vi "Invert if in Avoid Zone.vi"(7 "Avoid Zone (Unit Circle)":T4, 11 "Set Values":T1 {"Angle" scale format="%.3f"; "Velocity" scale=-1.0..1.0 scale format="%.1f"}) -> (2 "In Avoid Zone":bool, 3 "Set Values Out":T1 {"Angle" scale format="%.3f"; "Velocity" scale=-1.0..1.0 scale format="%.1f"})   [LabVIEW 2023, in "TShirtWork-SwerveDrive_ACT_ts.lvlib"]
uses:
  TShirtWork-SwerveDrive_ACT_ts.lvlib
  Shared Code/TypeDefs/Level_Velocity plus-minus 1.ctl
  Shared Code/TypeDefs/Dial_Compase heading unit circle CCW positive.ctl
  Shared Code/TypeDefs/Cluster_Module Velocity-Direction-Rotations.ctl
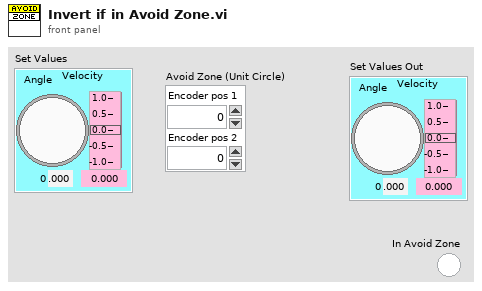
[diagram p1: front panel]
types:
  T1 = typedef "Cluster_Module Velocity-Direction-Rotations.ctl" = cluster{"Velocity":T2, "Angle":T3, "Rotations Count":dbl}
  T2 = typedef "Level_Velocity plus-minus 1.ctl" = dbl
  T3 = typedef "Dial_Compase heading unit circle CCW positive.ctl" = dbl
  T4 = cluster{"Encoder pos 1":dbl, "Encoder pos 2":dbl}
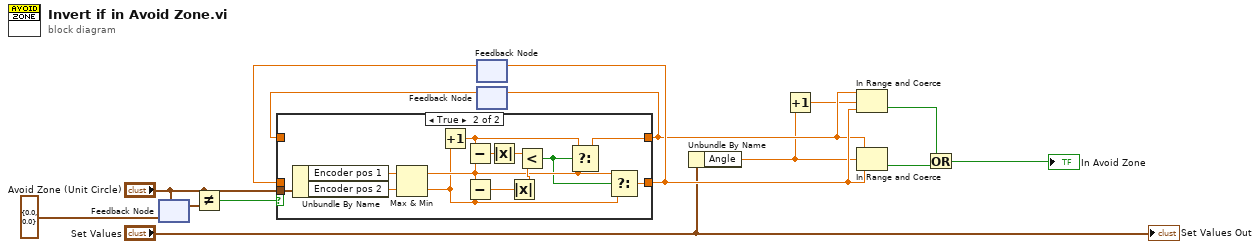
[diagram p0: block diagram]
diagram:
  n1 = feedback-in #1("Avoid Zone (Unit Circle)") -> ()
  n2 = feedback #1(T4 {"Encoder pos 1"=0.0, "Encoder pos 2"=0.0} ("Avoid Zone (Unit Circle)")) -> (w13:T4)
  n3 = Not Equal?(x="Avoid Zone (Unit Circle)", y=w13) -> (x != y?=w11:bool)
  n4 = feedback #2() -> (w9:dbl)  [unwired: 1 in]
  n5 = feedback #3() -> (w10:dbl)  [unwired: 1 in]
  n6 = case shown="True" w11 {
    tunnel: [w16 w20] -> w6
    tunnel: [w15 w19] -> w7
    tunnel: "Avoid Zone (Unit Circle)" -> [_ w17]
    tunnel: w10 -> [w16 _]
    tunnel: w9 -> [w15 _]
    frame False {
    }
    frame True {
      n7 = Unbundle By Name(w17) -> ("Encoder pos 1"=w29:dbl, "Encoder pos 2"=w28:dbl)
      n8 = Max & Min(x=w29, y=w28) -> (max(x,y)=w22:dbl, min(x,y)=w21:dbl)
      n9 = Increment(x=w21) -> (x+1=w23:dbl)
      n10 = Subtract(x=w23, y=w22) -> (x-y=w27:dbl)
      n11 = Subtract(x=w22, y=w21) -> (x-y=w26:dbl)
      n12 = Absolute Value(x=w27) -> (abs(x)=w25:dbl)
      n13 = Absolute Value(x=w26) -> (abs(x)=w24:dbl)
      n14 = Less?(x=w25, y=w24) -> (x < y?=w18:bool)
      n15 = Select(t=w23, s=w18, f=w22) -> (s? t:f=w20:dbl)
      n16 = Select(t=w22, s=w18, f=w21) -> (s? t:f=w19:dbl)
    }
  }
  n17 = feedback-in #2(w7) -> ()
  n18 = feedback-in #3(w6) -> ()
  n19 = Unbundle By Name("Set Values") -> ("Angle"=w5:T3)
  n20 = Increment(x=w5) -> (x+1=w4:T3)
  n21 = In Range and Coerce(upper limit=w6, x=w4, lower limit=w7) -> (In Range?=w2:bool)  [unwired: 1 out]
  n22 = In Range and Coerce(upper limit=w6, x=w5, lower limit=w7) -> (In Range?=w14:bool)  [unwired: 1 out]
  n23 = Or(x=w2, y=w14) -> (x .or. y?=→"In Avoid Zone":bool)
  "Set Values Out" <- "Set Values"
